vi "WPI_CameraBackground Loop_EDIT.vi"(0 "CameraDevRef":T1, 1 "CameraDevRef 2":T1) -> ()   [LabVIEW 2015]
doc: "This VI acquires the image buffer from the camera MJPG stream at the configured fps rate. It notifies any waiting VIs and allows them to pick up the latest image. This allows the camera and robot vision loop to run at different rates. The 1011, camera is far more efficient using MJPGs, and generally, this is probably the better choice for the camera loop.\n \nThis software is licensed. Open the labview\\readme\\WPI Robotics Library Open Source License.txt file for more information."
uses:
  <vilib>/Rock Robotics/WPI/Camera/WPI_CameraDevRef.ctl
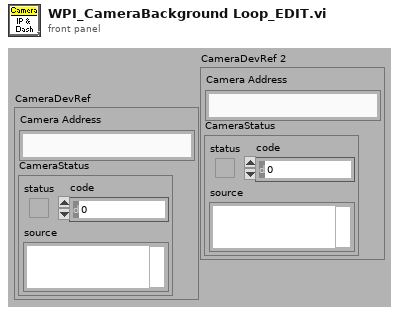
[diagram p1: front panel]
types:
  T1 = typedef "WPI_CameraDevRef.ctl" = cluster{"Camera Address":string, "CameraStatus":errorcluster}
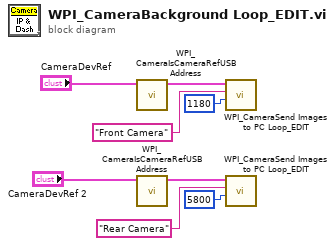
[diagram p0: block diagram]
diagram:
  n1 = call <vilib>:"WPI_CameraIsCameraRefUSBAddress.vi"("CameraDevRef"="CameraDevRef") -> ("CameraDevRef out"=w6:T1)  [unwired: 7 in, 3 out]
  n2 = call <vilib>:"WPI_CameraIsCameraRefUSBAddress.vi"("CameraDevRef"="CameraDevRef 2") -> ("CameraDevRef out"=w5:T1)  [unwired: 7 in, 3 out]
  n3 = call "WPI_CameraSend Images to PC Loop_EDIT.vi"("port"=u16 1180, "Image Name"="Front Camera", "CameraDevRef"=w6) -> ()  [unwired: 9 in]
  n4 = call "WPI_CameraSend Images to PC Loop_EDIT.vi"("port"=u16 5800, "Image Name"="Rear Camera", "CameraDevRef"=w5) -> ()  [unwired: 9 in]
